vi "BAP3B.vi"(0 "Header Comments":string="This is a C(T) experiment being done in Physics 350.\r\nIt records the decay response of an RC circuit where the capacitance is a strong function of temperature.", 5 "Temperature Control Parameters":T2={"Start Temp"=30.0, "Temp Step"=5.0, "End Temp"=80.0} {"End Temp" format="%.2f"; "Temp Step" format="%.2f"; "Start Temp" format="%.2f"}, 9 "Timing Control Parameters":T1={"N cycles for averaging"=10, "N points per measurment"=1000, "Measurment time interval"=2e-05} {"Measurment time interval" format="%.2e"}, 11 "error in":errorcluster) -> (4 "data file path out":path, 6 "Temp Array":dbl[](array[numeric]), 10 "Timing Control Parameters out":T1={"N cycles for averaging"=10, "N points per measurment"=1000, "Measurment time interval"=2e-05} {"Measurment time interval" format="%.2e"}, 15 "error out":errorcluster)   [LabVIEW 2014]
doc: "BAP3B\n\nInputs Temperature and Timing Control Parameters from front panel or from a file and displays header comments, file header with labels for corresponding data, and gives the option of creating a data before exiting. The Proeed and Auto Launch Viewer are indicators utilized in upcoming projects.\n\nError input and output is applied. \n\nBeverly Abadines\nPHY 350\nBAP3B"
uses:
  C:/Users/Beverly/Documents/LabVIEW Data/Phy_350/PHY_350/Projects/P3 R/P3 start/typedefs/temp control params.ctl
  C:/Users/Beverly/Documents/LabVIEW Data/Phy_350/PHY_350/Projects/P3 R/P3 start/typedefs/time control params.ctl
panel:
  out "Warning":bool=TRUE
  out "Proceed":bool
  out "Auto Launch Data Viewer at End":bool=TRUE
  in  "reload parameters":bool
  in  "exit":bool
  in  "create file and proceed":bool
  out "File Header":string="This is a C(T) experiment being done in Physics 350.\r\nIt records the decay response of an RC circuit where the capacitance is a strong function of temperature.\n\n2/14/2007\n1:53 PM\r\n\r\nStart temp = 30.0\r\nTemp step = 10.0\r\nEnd temp = 80.0\r\nNum temps = 6\r\nNum avg cycles = 10\r\nNum points per meas = 1000\r\nMeas time interval = 2.00E-5\n\nDDD\n\n"
  out "N temps":i32=6
  in  "Auto Launch Data Viewer at End":bool=TRUE
  # "Beverly Abadines\nPhys 350"
  # "BAP3B"
  # "P350 C(T) Experimental Initialization"
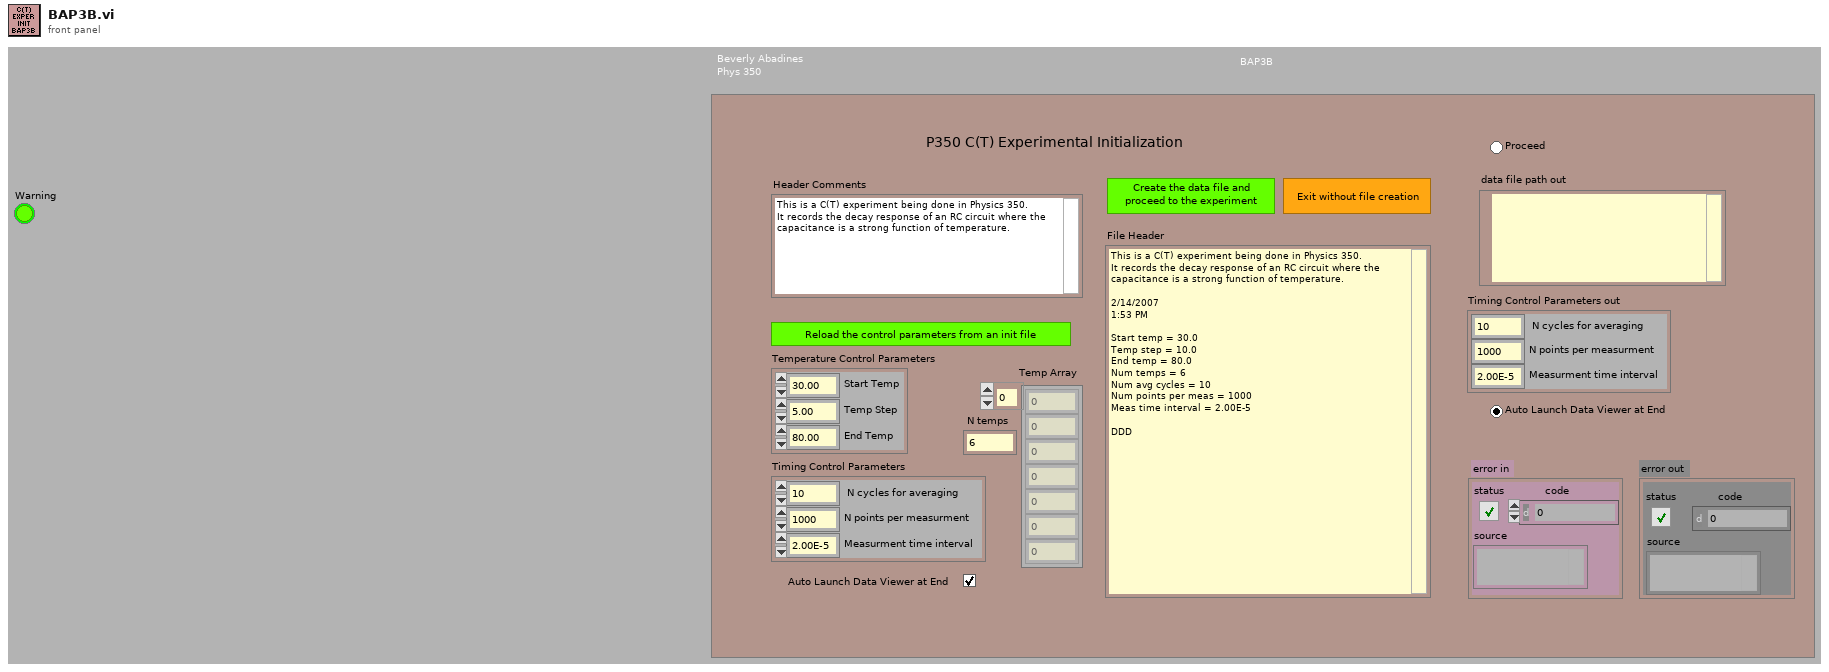
[diagram p1: front panel]
types:
  T1 = typedef "time control params.ctl" = cluster{"N cycles for averaging":i32, "N points per measurment":i32, "Measurment time interval":dbl}
  T2 = typedef "temp control params.ctl" = cluster{"Start Temp":dbl, "Temp Step":dbl, "End Temp":dbl}
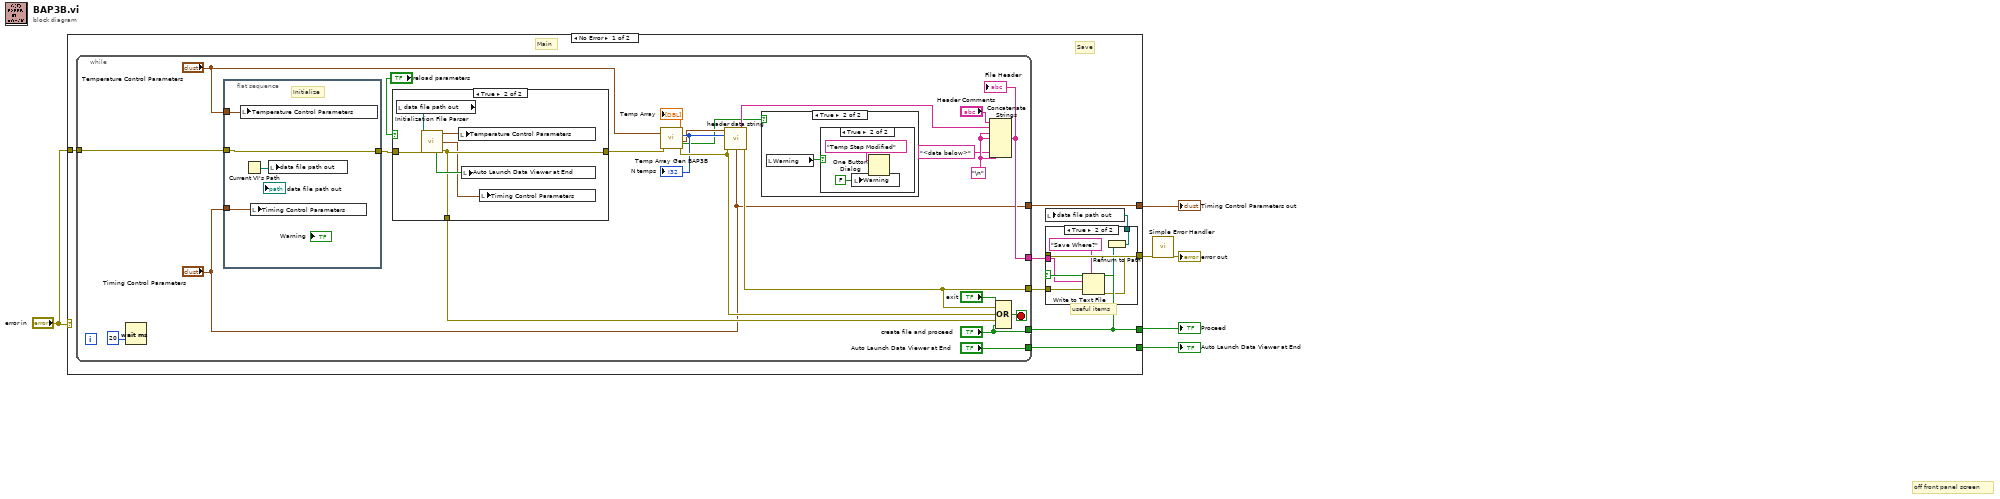
[diagram p0: block diagram]
diagram:
  # "useful items"
  # "off front panel screen"
  n1 = case shown="No Error" "error in" {
    selector: "error in" -> [_ w58]
    tunnel: "error in" -> [w8 _]
    tunnel: [w12 w58] -> w6
    tunnel: [w9 _] -> w2
    tunnel: [w10 _] -> w3
    tunnel: [w7 _] -> w1
    frame No Error {
      # "Save"
      # "Main"
      n2 = while {
        tunnel: [w28] -> w13
        tunnel: [w42] -> w14
        tunnel: ["create file and proceed"] -> w9
        tunnel: ["Auto Launch Data Viewer at End"] -> w10
        tunnel: w8 -> [w33]
        tunnel: ["Timing Control Parameters"] -> w7
        stop <- w41 stop-if-true
        w37 = "\n"
        n3 = Wait (ms)(milliseconds to wait=u32 20) -> ()  [unwired: 1 out]
        n4 = flat-sequence {
          tunnel: "Timing Control Parameters" -> [w50]
          tunnel: "Temperature Control Parameters" -> [w49]
          tunnel: w33 -> [w48]
          tunnel: [w48] -> w32
          frame #0 {
            # "Initialize"
            n5 = local write "Temperature Control Parameters"(w49) -> ()
            n6 = Current VI's Path() -> (path=w51:path)
            n7 = local write "Timing Control Parameters"(w50) -> ()
            n8 = local write "data file path out"(w51) -> ()
          }
        }
        n9 = case shown="True" "reload parameters" {
          tunnel: [_ w56] -> w30
          tunnel: [_ w56] -> w39
          tunnel: w32 -> [_ w52]
          frame False {
          }
          frame True {
            n10 = local read "data file path out"() -> (w55:path)
            n11 = call "Initialization File Parser.vi"("path in"=w55, "error in"=w52) -> ("Auto Launch Data Viewer at End"=w57:bool, "temp control parameters"=w53:T2, "time control parameters"=w54:T1, "error out"=w56:errorcluster)  [unwired: 9 in, 1 out]
            n12 = local write "Temperature Control Parameters"(w53) -> ()
            n13 = local write "Auto Launch Data Viewer at End"(w57) -> ()
            n14 = local write "Timing Control Parameters"(w54) -> ()
          }
        }
        n15 = call "Temp Array Gen BAP3B.vi"("error in (no error)"=w30, "Temperature Control Parameters"="Temperature Control Parameters") -> ("error out"=w29:errorcluster, "Temperature Control Parameters Out"=w23:T2, "N Temps"=w26:i32, "Temp Array"=→"Temp Array":dbl[], "Warning"=w22:bool)  [unwired: 5 in]
        "N temps" <- w26
        n16 = call "header data string.vi"("Temperature Control Parameters"=w23, "N temps"=w26, "error in (no error)"=w29, "Timing Control Parameters"="Timing Control Parameters") -> ("Header string component"=w27:string, "error out"=w28:errorcluster)  [unwired: 10 in]
        n17 = case shown="True" w22 {
          frame False {
          }
          frame True {
            n18 = local read "Warning"() -> (w45:bool)
            n19 = case shown="True" w45 {
              frame False {
              }
              frame True {
                n20 = local write "Warning"(FALSE ("Warning")) -> ()
                n21 = One Button Dialog(message="Temp Step Modified") -> ()  [unwired: 1 in, 1 out]
              }
            }
          }
        }
        n22 = Concatenate Strings("Header Comments", w27, w37, w37, "<data below>", w37, w37) -> (w42:string)
        "File Header" <- w42
        n23 = Compound Arithmetic op=OR("exit", w28, w29, w39, "create file and proceed") -> (w41:bool)
      }
      n24 = case shown="True" w9 {
        tunnel: [w15 w20] -> w12
        tunnel: w13 -> [w15 w19]
        tunnel: [_ w18] -> w11
        tunnel: w14 -> [_ w17]
        frame False {
        }
        frame True {
          n25 = Write to Text File(prompt (Choose or enter file path)="Save Where?", text=w17, error in=w19) -> (refnum out=w21:refnum<file>, error out=w20:errorcluster)  [unwired: 1 in, 1 out]
          n26 = Refnum to Path(1:w21) -> (0:w18:path)
        }
      }
      n27 = local write "data file path out"(w11) -> ()
    }
    frame Error {
    }
  }
  "Timing Control Parameters out" <- w1
  "Auto Launch Data Viewer at End" <- w3
  "Proceed" <- w2
  n28 = call <vilib>:"Simple Error Handler.vi"("error in (no error)"=w6) -> ("error out"=→"error out":errorcluster)  [unwired: 4 in, 4 out]
